vi "Auto Indexing.vi"() -> ()   [LabVIEW 2020]
panel:
  in  "stop":bool
  out "Index":i32
  out "Index value":dbl
  in  "5 element array":dbl[](array[numeric])
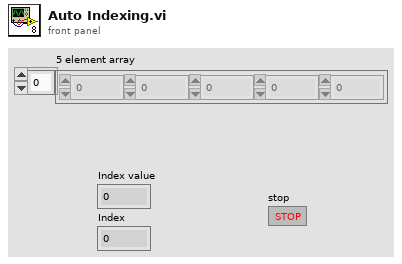
[diagram p1: front panel]
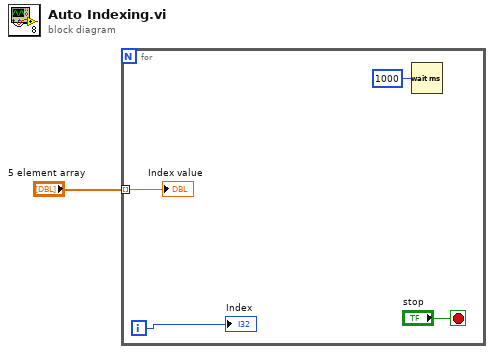
[diagram p0: block diagram]
diagram:
  n1 = for {
    tunnel: "5 element array" -> [w5] mode=indexing
    i -> [w2]
    stop <- "stop" stop-if-true
    n2 = Wait (ms)(milliseconds to wait=u32 1000) -> ()  [unwired: 1 out]
    "Index value" <- w5
    "Index" <- w2
  }
